vi "startUp.vi"(8 "error in (no error)":errorcluster, 11 "ImageStreamViewer in":refnum<class "ImageStreamViewer.lvclass">) -> (0 "error out":errorcluster, 3 "ImageStreamViewer out":refnum<class "ImageStreamViewer.lvclass">)   [LabVIEW 2011, in "Views.lvlib" / "Camera.lvlib" / "ImageStreamViewer.lvclass"]
uses:
  ImageStreamViewer.lvclass
  Tools/ImageProcessor/ImageAnalyser/FluorescenceLiveAnalyser/FluorescenceLiveAnalyser.lvclass
  ImageStreamViewer.lvclass/ImageStreamViewer.ctl
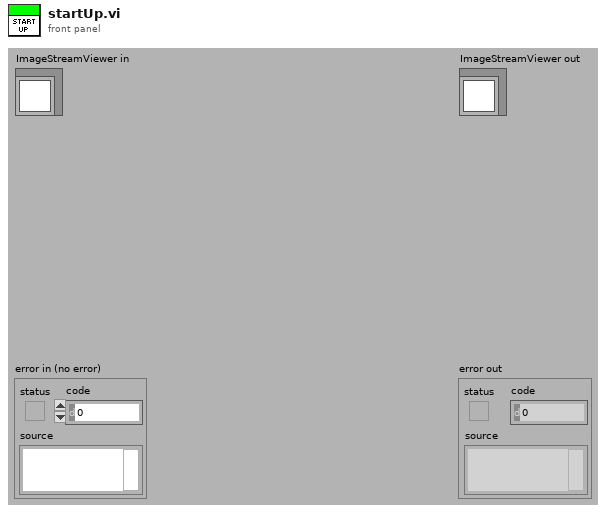
[diagram p1: front panel]
types:
  T1 = typedef "Image Type" = u32
  T2 = typedef "IMAQ Image.ctl" = refnum<image>
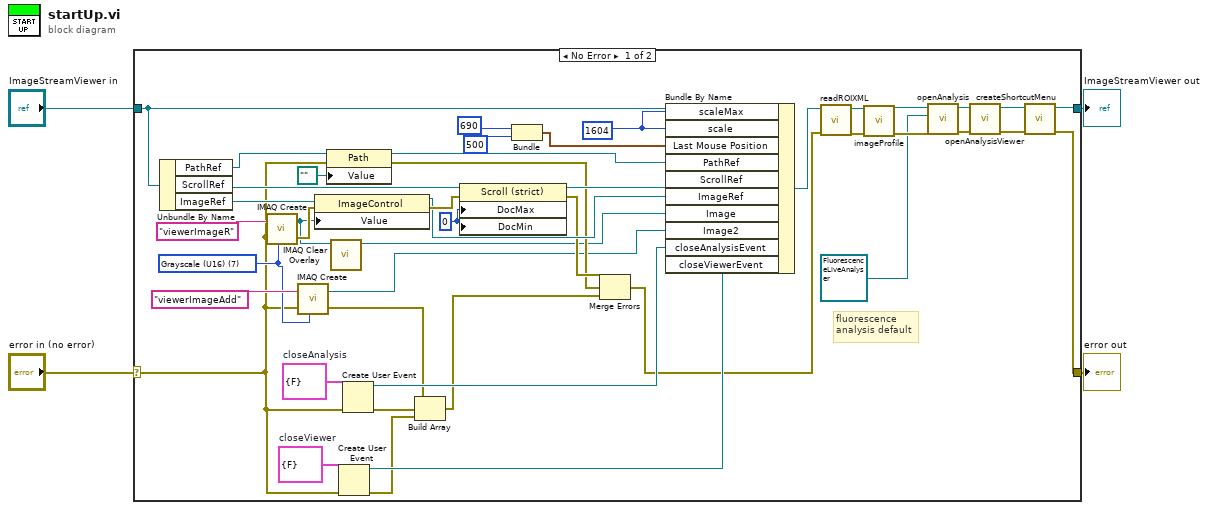
[diagram p0: block diagram]
diagram:
  n1 = case shown="No Error" "error in (no error)" {
    selector: "error in (no error)" -> [w12 w51]
    tunnel: [w5 w51] -> w3
    tunnel: [w6 w50] -> w1
    tunnel: "ImageStreamViewer in" -> [w41 w50]
    frame No Error {
      w9 = 1604
      w30 = cluster{"close":bool} {"close"=FALSE}  # closeViewer
      w35 = cluster{"close":bool} {"close"=FALSE}  # closeAnalysis
      w44 = 0
      w13 = T1 7 items=["Grayscale (U8)", "Grayscale (I16)", "Grayscale (SGL)", "Complex (CSG)", "RGB (U32)", "HSL (U32)", "RGB (U64)", "Grayscale (U16)"] ("Image Type")
      # "fluorescence \nanalysis default"
      n2 = Unbundle By Name(w41) -> ("PathRef"=w40:refnum<vi>, "ScrollRef"=w46:refnum<vi>, "ImageRef"=w47:refnum<vi>)
      n3 = call "IMAQ Create"("Image Name"="viewerImageR", "Image Type"=w13, "error in (no error)"=w12) -> ("New Image"=w17:T2, "error out"=w48:errorcluster)  [unwired: 2 in]
      n4 = call "IMAQ Create"("Image Name"="viewerImageAdd", "Image Type"=w13, "error in (no error)"=w12) -> ("New Image"=w10:T2, "error out"=w11:errorcluster)  [unwired: 2 in]
      n5 = property class="ImageControl"(reference=w47, error in=w48, "Value"=w17) -> (reference out=w42:refnum<vi>, error out=w45:errorcluster)
      n6 = property class="Path"(reference=w40, error in=w12, "Value"=path "") -> (reference out=w36:refnum<vi>, error out=w37:errorcluster)
      n7 = call "IMAQ Clear Overlay"("Image"=w17) -> ("Image Out"=w16:T2)  [unwired: 9 in, 1 out]
      n8 = Create User Event(user event datatype=w30, error in=w12) -> (user event=w29:refnum<user-event>, error out=w27:errorcluster)
      n9 = Create User Event(user event datatype=w35, error in=w12) -> (user event=w34:refnum<user-event>, error out=w28:errorcluster)
      n10 = Build Array(w11, w28, w27) -> (w26:errorcluster[])
      n11 = property class="Scroll (strict)"(reference=w46, error in=w45, "DocMax"=w44, "DocMin"=w44) -> (reference out=w43:refnum<vi>, error out=w38:errorcluster)
      n12 = Bundle(690, 500) -> (w31:cluster{i32, i32})  [unwired: 1 in]
      n13 = Merge Errors(w38, w37, w26) -> (w22:errorcluster)
      n14 = Bundle By Name(cluster=w41, "scaleMax"=w9, "scale"=w9, "Last Mouse Position"=w31, "PathRef"=w36, "ScrollRef"=w43, "ImageRef"=w42, "Image"=w16, "Image2"=w10, "closeAnalysisEvent"=w34, "closeViewerEvent"=w29) -> (w23:refnum<class "ImageStreamViewer.lvclass">)
      n15 = call "readROIXML.vi"("error in (no error)"=w22, "ImageStreamViewer in"=w23) -> ("error out"=w20:errorcluster, "ImageStreamViewer out"=w21:refnum<class "ImageStreamViewer.lvclass">)  [unwired: 8 in]
      n16 = call "imageProfile.vi"("error in (no error)"=w20, "ImageStreamViewer in"=w21) -> ("error out"=w18:errorcluster, "ImageStreamViewer out"=w19:refnum<class "ImageStreamViewer.lvclass">)  [unwired: 8 in]
      n17 = call "openAnalysis.vi"("error in (no error)"=w18, "ImageAnalyser"=refnum<class "FluorescenceLiveAnalyser.lvclass"> refnum ("Tools.lvlib:Imaging.lvlib:FluorescenceLiveAnalyser.lvclass"), "ImageStreamViewer in"=w19) -> ("error out"=w24:errorcluster, "ImageStreamViewer out"=w25:refnum<class "ImageStreamViewer.lvclass">)  [unwired: 7 in]
      n18 = call "openAnalysisViewer.vi"("error in (no error)"=w24, "ImageStreamViewer in"=w25) -> ("error out"=w7:errorcluster, "ImageStreamViewer out"=w8:refnum<class "ImageStreamViewer.lvclass">)  [unwired: 8 in]
      n19 = call "createShortcutMenu.vi"("error in (no error)"=w7, "ImageStreamViewer in"=w8) -> ("error out"=w5:errorcluster, "ImageStreamViewer out"=w6:refnum<class "ImageStreamViewer.lvclass">)  [unwired: 8 in]
    }
    frame Error {
    }
  }
  "error out" <- w3
  "ImageStreamViewer out" <- w1
